vi "Draw Fixed Wheel.vi"(6 "wheel state":T1, 7 "picture info":T3={"picture size"={"Width"=500, "Height"=500}, "pixels per unit"=10.0}, 8 "error in (no error)":errorcluster, 9 "draw wheel options":T2={"global wheel position"={"x"=0.0, "y"=0.0}, "wheel frame angle (rad)"=0.0, "color (black)"=0, "draw wheel state"=FALSE, "draw forward velocity"=FALSE, "velocity scale"=16711680.0, "velocity color (red)"=16711680}, 10 "picture in":picture, 11 "wheel in":refnum<class "NI_Robotics_Wheel.lvclass">) -> (0 "error out":errorcluster, 2 "picture out":picture, 3 "wheel out":refnum<class "NI_Robotics_Wheel.lvclass">)   [LabVIEW 2017, in "NI_Robotics_Steering Picture.lvlib"]
uses:
  <vilib>/robotics/Utilities/Visualization/Steering Visualization/Steering Picture/NI_Robotics_Steering Picture.lvlib
  <vilib>/robotics/Steering/Wheel/NI_Robotics_Wheel.lvclass
  <vilib>/robotics/Utilities/Visualization/Steering Visualization/Steering Picture/Picture Info.ctl
  <vilib>/Utility/miscctls.llb/LVBoundsTypeDef.ctl
  <vilib>/robotics/Utilities/Visualization/Steering Visualization/Steering Picture/Draw Wheel Options.ctl
  <vilib>/robotics/Steering/Wheel/Wheel State.ctl
  <vilib>/Analysis/coordinate.llb/2D Cartesian Coordinate Rotation.vi
  <vilib>/Analysis/coordinate.llb/2D Cartesian Coordinate Rotation (Array).vi
  <vilib>/robotics/Utilities/Visualization/Steering Visualization/Steering Picture/Global Position to Pixel.vi
  <vilib>/Analysis/coordinate.llb/Angle Rotation.vi
  <vilib>/Analysis/coordinate.llb/Angle Rotation (scalar).vi
  <vilib>/Analysis/coordinate.llb/Wrap Angle (scalar).vi
  <vilib>/picture/picture.llb/Draw Line.vi
  <vilib>/picture/picture.llb/Move Pen.vi
  <vilib>/picture/picture.llb/Draw Point.vi
  <vilib>/picture/picture.llb/Draw Multiple Lines.vi
  <vilib>/robotics/Steering/Wheel/Get Fixed Wheel Information.vi
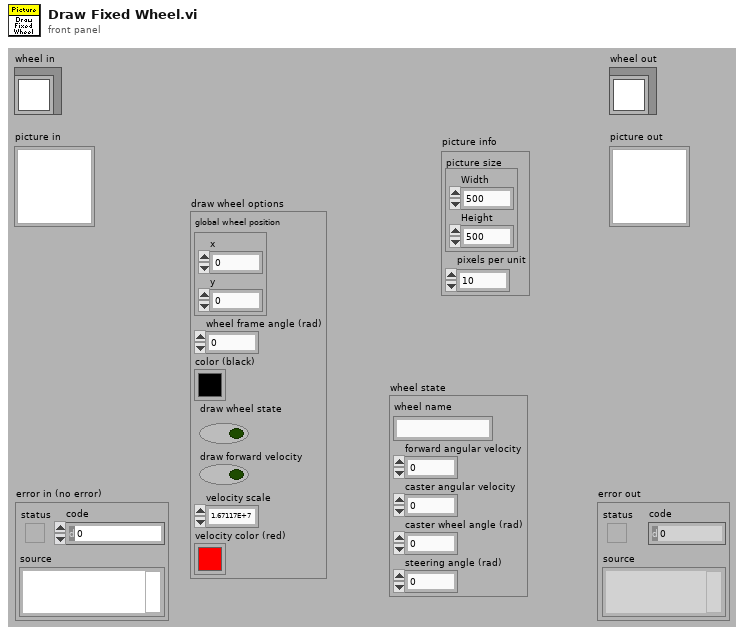
[diagram p1: front panel]
types:
  T1 = typedef "NI_Robotics_Wheel.lvclass/Wheel State.ctl" = cluster{"wheel name":string, "forward angular velocity":dbl, "caster angular velocity":dbl, "caster wheel angle (rad)":dbl, "steering angle (rad)":dbl}
  T2 = typedef "NI_Robotics_Steering Picture.lvlib/Draw Wheel Options.ctl" = cluster{"global wheel position":cluster{"x":dbl, "y":dbl}, "wheel frame angle (rad)":dbl, "color (black)":u32, "draw wheel state":bool, "draw forward velocity":bool, "velocity scale":dbl, "velocity color (red)":u32}
  T3 = typedef "NI_Robotics_Steering Picture.lvlib/Picture Info.ctl" = cluster{"picture size":T4, "pixels per unit":dbl}
  T4 = typedef "LVBoundsTypeDef.ctl" = cluster{"Width":u32, "Height":u32}
  T5 = typedef "NI_Robotics_Wheel.lvclass/Wheel Parameters.ctl" = cluster{"wheel radius":dbl, "gear ratio":dbl, "forward rotation direction":T6}
  T6 = typedef "NI_Robotics_Wheel.lvclass/Rotation Direction.ctl" = u16
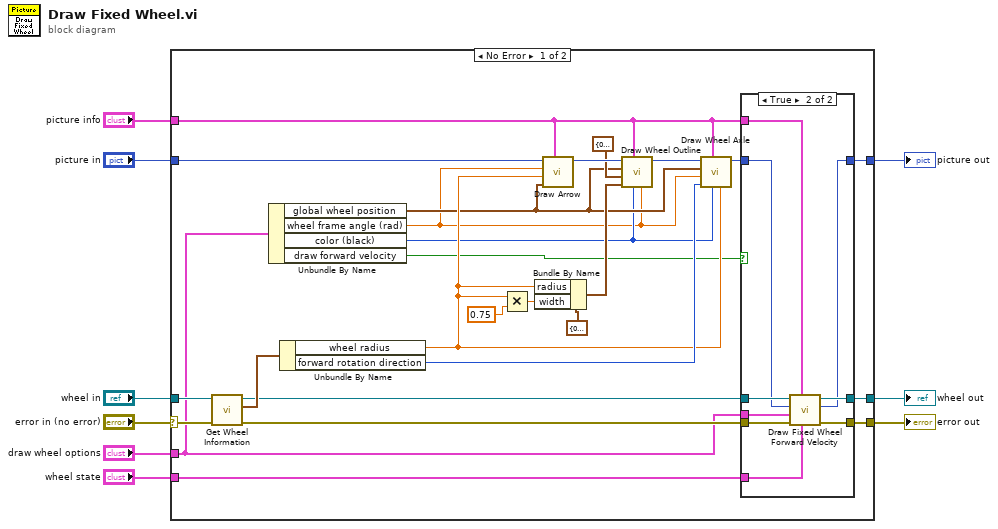
[diagram p0: block diagram]
diagram:
  n1 = case shown="No Error" "error in (no error)" {
    selector: "error in (no error)" -> [w34 w50]
    tunnel: [w16 w50] -> w9
    tunnel: "wheel in" -> [w35 w48]
    tunnel: "picture in" -> [w32 w49]
    tunnel: [w14 w49] -> w6
    tunnel: [w18 w48] -> w5
    tunnel: "picture info" -> [w12 _]
    tunnel: "draw wheel options" -> [w10 _]
    tunnel: "wheel state" -> [w11 _]
    frame No Error {
      n2 = call-poly <vilib>:"Get Wheel Information.vi"("error in (no error)"=w34, "wheel in"=w35) -> ("error out"=w17:errorcluster, "wheel parameters"=w33:T5, "wheel out"=w19:refnum<class "NI_Robotics_Wheel.lvclass">)  [unwired: 5 in, 2 out]
      n3 = Unbundle By Name(w10) -> ("global wheel position"=w22:cluster{"x":dbl, "y":dbl}, "wheel frame angle (rad)"=w20:dbl, "color (black)"=w21:u32, "draw forward velocity"=w13:bool)
      n4 = Unbundle By Name(w33) -> ("wheel radius"=w23:dbl, "forward rotation direction"=w31:T6)
      n5 = Multiply(x=w23, y=0.75) -> (x*y=w24:dbl)
      n6 = Bundle By Name(cluster=cluster{"radius":dbl, "width":dbl} {"radius"=0.0, "width"=0.0} ("size"), "radius"=w23, "width"=w24) -> (w26:cluster{"radius":dbl, "width":dbl})
      n7 = call <vilib>:"Draw Arrow.vi"("picture info"=w12, "global base position"=w22, "length"=w23, "wheel frame angle (rad)"=w20, "picture in"=w32) -> ("picture out"=w30:picture)  [unwired: 6 in]
      n8 = call <vilib>:"Draw Wheel Outline.vi"("angle (rad)"=w20, "color (black)"=w21, "picture info"=w12, "size"=w26, "offset from center"=cluster{"x":dbl, "y":dbl} {"x"=0.0, "y"=0.0}, "global wheel position"=w22, "picture in"=w30) -> ("picture out"=w29:picture)  [unwired: 4 in]
      n9 = call <vilib>:"Draw Wheel Axle.vi"("length"=w23, "color (black)"=w21, "picture info"=w12, "rotation direction"=w31, "wheel frame angle (rad)"=w20, "global wheel position"=w22, "picture in"=w29) -> ("picture out"=w15:picture)  [unwired: 4 in]
      n10 = case shown="True" w13 {
        tunnel: w19 -> [w37 w47]
        tunnel: [w37 w46] -> w18
        tunnel: w17 -> [w36 w45]
        tunnel: [w36 w44] -> w16
        tunnel: w15 -> [w38 w43]
        tunnel: [w38 w42] -> w14
        tunnel: w12 -> [_ w41]
        tunnel: w11 -> [_ w40]
        tunnel: w10 -> [_ w39]
        frame False {
        }
        frame True {
          n11 = call <vilib>:"Draw Fixed Wheel Forward Velocity.vi"("wheel state"=w40, "picture info"=w41, "error in (no error)"=w45, "draw wheel options"=w39, "picture in"=w43, "wheel in"=w47) -> ("error out"=w44:errorcluster, "picture out"=w42:picture, "wheel out"=w46:refnum<class "NI_Robotics_Wheel.lvclass">)  [unwired: 3 in]
        }
      }
    }
    frame Error {
    }
  }
  "error out" <- w9
  "wheel out" <- w5
  "picture out" <- w6
